vi "ViTrig.vi"(5 "Vi Trigger":bool=TRUE, 8 "error in":errorcluster, 11 "FPGA VI Reference":T1) -> (0 "error out":errorcluster, 3 "FPGA VI Reference Out":T1)   [LabVIEW 2020]
uses:
  DigiFPGARef.ctl
  <vilib>/Utility/error.llb/Error Cluster From Error Code.vi
  <vilib>/rvi/errors/niLvFpgaAdjustHostInterfaceError.vi
  <vilib>/rvi/interface/nirviReadWriteControl/nirviReadWriteControl.xnode
  NiFpgaLv.dll
  <vilib>/rvi/interface/Simulation/niFpgaSimulationCallBeginRW.vi
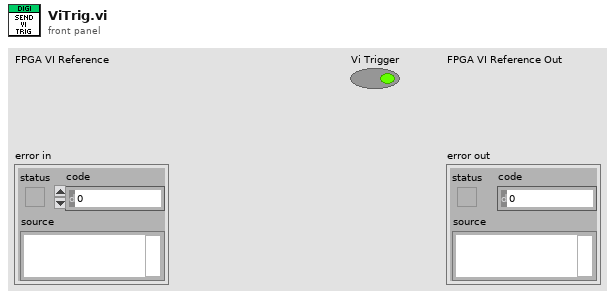
[diagram p1: front panel]
types:
  T1 = typedef "DigiFPGARef.ctl" = refnum<k20>
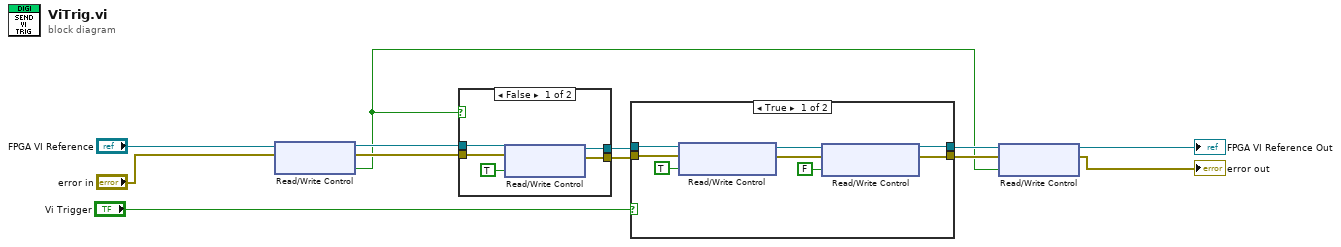
[diagram p0: block diagram]
diagram:
  n1 = xnode "Read/Write Control"("FPGA VI Reference In"="FPGA VI Reference", "error in"="error in") -> ("FPGA VI Reference Out"=w5:T1, "error out"=w4:errorcluster, "vi/nGenTrig"=w1:bool)
  n2 = case shown="False" w1 {
    tunnel: [w17 w19] -> w12
    tunnel: [w16 w18] -> w11
    tunnel: w5 -> [w14 w19]
    tunnel: w4 -> [w13 w18]
    frame False {
      n3 = xnode "Read/Write Control"("FPGA VI Reference In"=w14, "error in"=w13, "vi/nGenTrig"=TRUE) -> ("FPGA VI Reference Out"=w17:T1, "error out"=w16:errorcluster)
    }
    frame True {
    }
  }
  n4 = case shown="True" "Vi Trigger" {
    tunnel: w12 -> [w27 w29]
    tunnel: w11 -> [w26 w28]
    tunnel: [w20 w29] -> w9
    tunnel: [w21 w28] -> w8
    frame True {
      n5 = xnode "Read/Write Control"("FPGA VI Reference In"=w27, "error in"=w26, "TrigIn Simulate"=TRUE ("Arm Trigger")) -> ("FPGA VI Reference Out"=w23:T1, "error out"=w22:errorcluster)
      n6 = xnode "Read/Write Control"("FPGA VI Reference In"=w23, "error in"=w22, "TrigIn Simulate"=FALSE ("Arm Trigger")) -> ("FPGA VI Reference Out"=w20:T1, "error out"=w21:errorcluster)
    }
    frame False {
    }
  }
  n7 = xnode "Read/Write Control"("FPGA VI Reference In"=w9, "error in"=w8, "vi/nGenTrig"=w1) -> ("FPGA VI Reference Out"=→"FPGA VI Reference Out":T1, "error out"=→"error out":errorcluster)
